vi "Test_WriteValue_CheckItemNames_NamesUpdated.vi"(8 "error in (no error)":errorcluster, 11 "TestCase in":refnum<class "TestMCListboxItemNamesBinding.lvclass">) -> (0 "error out":errorcluster, 3 "TestCase out":refnum<class "TestMCListboxItemNamesBinding.lvclass">)   [LabVIEW 2017, in "TestMCListboxItemNamesBinding.lvclass"]
uses:
  TestMCListboxItemNamesBinding.lvclass
  Source/Concrete/MCListboxItemNamesBinding/MCListboxItemNamesBinding.lvclass/MCListboxItemNamesBinding.ctl
  Source/Concrete/MCListboxItemNamesBinding/MCListboxItemNamesBinding.lvclass
  C:/Git/composed-transport/Source/ITransport/ITransport.lvclass
  <vilib>/Utility/error.llb/Error Cluster From Error Code.vi
  Source/ITransport/ITransport.lvclass
panel:
  in  "Multicolumn Listbox":i32(listbox)
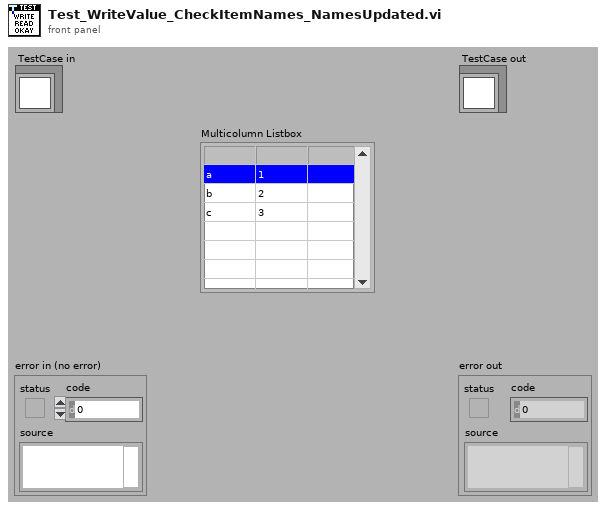
[diagram p1: front panel]
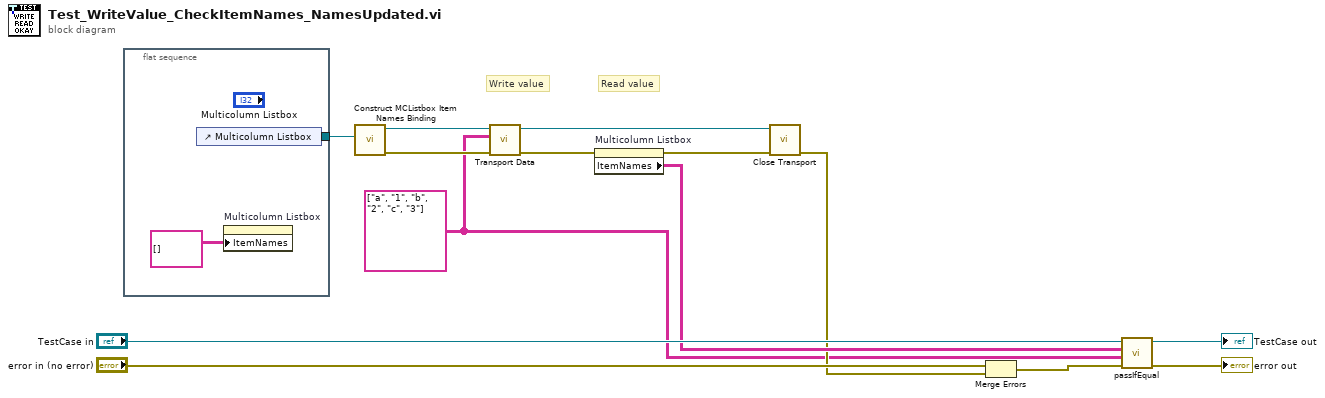
[diagram p0: block diagram]
diagram:
  w1 = string[][] [["a", "1"], ["b", "2"], ["c", "3"]]
  # "Read value"
  # "Write value"
  n1 = flat-sequence {
    tunnel: [w16] -> w6
    frame #0 {
      n2 = control-ref of="Multicolumn Listbox"() -> (w16:refnum<vi>)
      n3 = property on="Multicolumn Listbox" class="MCListbox (strict)"("ItemNames"=string[][] []) -> ()  [unwired: 2 in, 2 out]
    }
  }
  n4 = call "Construct MCListbox Item Names Binding.vi"("MCListbox Refnum"=w6) -> ("error out"=w8:errorcluster, "MCListboxItemNamesBinding"=w10:refnum<class "MCListboxItemNamesBinding.lvclass">)  [unwired: 9 in]
  n5 = call "Transport Data.vi"("error in (no error)"=w8, "Value"=w1, "ITransport in"=w10) -> ("error out"=w5:errorcluster, "ITransport out"=w7:refnum<class "MCListboxItemNamesBinding.lvclass">)  [unwired: 7 in]
  n6 = property on="Multicolumn Listbox" class="MCListbox (strict)"(error in=w5) -> (error out=w4:errorcluster, "ItemNames"=w3:string[][])  [unwired: 1 in, 1 out]
  n7 = call-dynamic "Close Transport.vi"("error in (no error)"=w4, "ITransport in"=w7) -> ("error out"=w2:errorcluster)  [unwired: 9 in]
  n8 = Merge Errors("error in (no error)", w2) -> (w9:errorcluster)
  n9 = call-dynamic "passIfEqual.vi"("error in (no error)"=w9, "y"=w1, "x"=w3, "TestCase in"="TestCase in") -> ("error out"=→"error out":errorcluster, "TestCase out"=→"TestCase out":refnum<class "TestMCListboxItemNamesBinding.lvclass">)  [unwired: 6 in]
